vi "Data Into Buffer.vi"(8 "error in (no error)":errorcluster, 9 "Current Through Diode":dbl, 10 "Voltage Across Diode":dbl, 11 "Top Level in":refnum<class "Top Level.lvclass">) -> (0 "error out":errorcluster, 3 "Top Level out":refnum<class "Top Level.lvclass">)   [LabVIEW 2021, in "Top Level.lvlib" / "Top Level.lvclass"]
uses:
  Top Level.lvclass
  Top Level.lvclass/Top Level.ctl
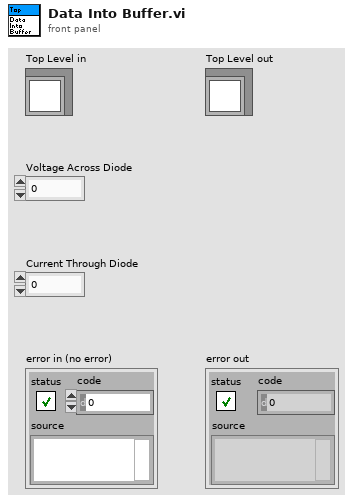
[diagram p1: front panel]
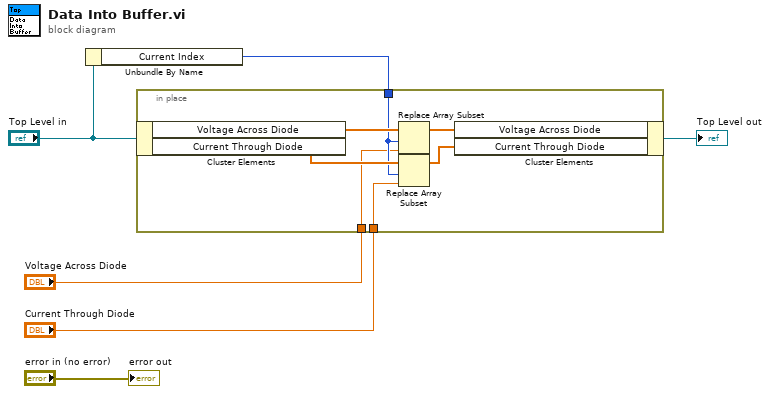
[diagram p0: block diagram]
diagram:
  n1 = Unbundle By Name("Top Level in") -> ("Current Index"=w5:i32)
  n2 = in-place {
    in-place-border: w5 -> [w9]
    in-place-border: "Voltage Across Diode" -> [w8]
    in-place-border: "Current Through Diode" -> [w7]
    n3 = in-place-cluster #1("Top Level in") -> ("Voltage Across Diode"=w13:dbl[], "Current Through Diode"=w11:dbl[])
    n4 = Replace Array Subset(array=w13, new element=w8, index=w9) -> (w12:dbl[])
    n5 = Replace Array Subset(array=w11, new element=w7, index=w9) -> (w10:dbl[])
    n6 = in-place-cluster #1("Voltage Across Diode"=w12, "Current Through Diode"=w10) -> (→"Top Level out":refnum<class "Top Level.lvclass">)
  }
  "error out" <- "error in (no error)"
